vi "Create Container if Unowned.vi"(8 "error in (no error)":errorcluster, 9 "Item Is Unowned?":bool, 10 "Create Unowned Container?":bool, 11 "Fully Qualified Name":string) -> (0 "error out":errorcluster, 3 "DGML Strings out":string[](array[string]))   [LabVIEW 2018, in "DGML creation.lvlib"]
uses:
  DGML Creation/DGML creation.lvlib
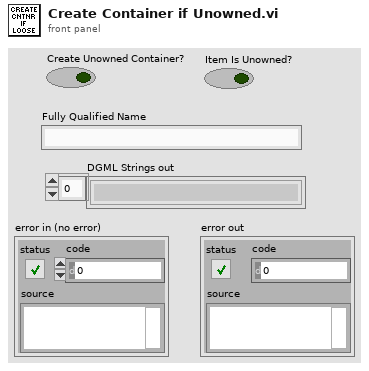
[diagram p1: front panel]
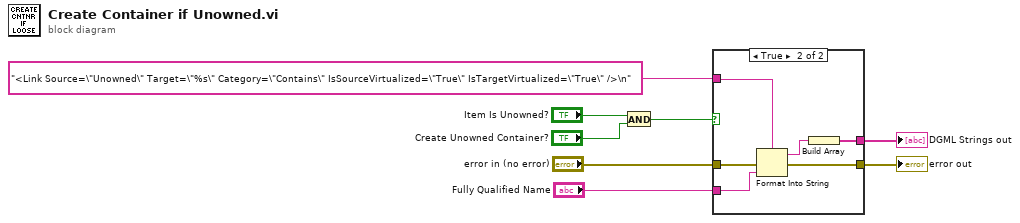
[diagram p0: block diagram]
diagram:
  n1 = And(x="Item Is Unowned?", y="Create Unowned Container?") -> (x .and. y?=w3:bool)
  n2 = case shown="True" w3 {
    tunnel: "<Link Source=\"Unowned\" Target=\"%s\" Category=\"Contains\" IsSourceVirtualized=\"True\" IsTargetVirtualized=\"True\" />\n" ("format string") -> [_ w11]
    tunnel: "Fully Qualified Name" -> [_ w10]
    tunnel: [_ w14] -> w1
    tunnel: "error in (no error)" -> [w9 w13]
    tunnel: [w9 w12] -> w6
    frame False {
    }
    frame True {
      n3 = Format Into String(format string=w11, error in=w13, w10) -> (resulting string=w15:string, error out=w12:errorcluster)  [unwired: 1 in]
      n4 = Build Array(w15) -> (w14:string[])
    }
  }
  "error out" <- w6
  "DGML Strings out" <- w1
